vi "TestArrays.vi"() -> ()   [LabVIEW 2010]
panel:
  in  "Array":u32[](array[numeric])
  out "Numeric 10":i32
  out "Numeric 9":i32
  out "Numeric 8":i32
  out "Numeric 7":i32
  out "Numeric 6":i32
  out "Numeric 5":i32
  out "Numeric 4":i32
  out "Numeric 3":i32
  out "Numeric 2":i32
  out "Numeric":i32
  out "element":dbl format="%.2f"
  in  "Array Size":i32
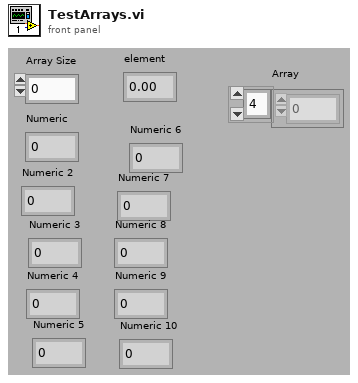
[diagram p1: front panel]
types:
  T1 = cluster{i32, i32, i32, i32, i32, i32, i32, i32, i32, i32}
  T2 = cluster{"[0]":i32, "[1]":i32, "[2]":i32, "[3]":i32, "[4]":i32, "[5]":i32, "[6]":i32, "[7]":i32, "[8]":i32}
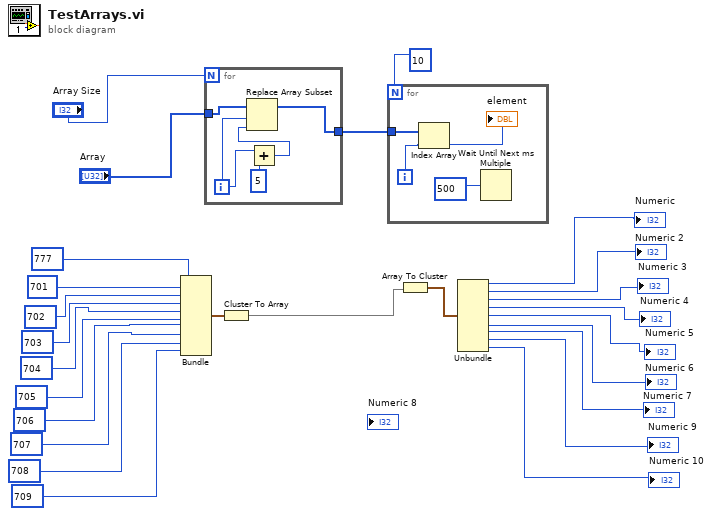
[diagram p0: block diagram]
diagram:
  n1 = Bundle(777, 701, 702, 703, 704, 705, 706, 707, 708, 709) -> (w6:T1)  [unwired: 1 in]
  n2 = for {
    N: "Array Size" -> [_]
    tunnel: "Array" -> [w31]
    tunnel: [w30] -> w2
    i -> [w28]
    n3 = Add(x=w28, y=u32 5) -> (x+y=w27:u32)
    n4 = Replace Array Subset(array=w31, new element=w27, index=w28) -> (w30:u32[])
  }
  n5 = Cluster To Array(cluster=w6) -> (array=w3:i32[])
  n6 = for {
    N: 10 -> [_]
    tunnel: w2 -> [w33]
    i -> [w35]
    n7 = Index Array(array=w33, index=w35) -> (element=→"element":u32)
    n8 = Wait Until Next ms Multiple(millisecond multiple=500) -> ()  [unwired: 1 out]
  }
  n9 = Array To Cluster(array=w3) -> (cluster=w26:T2)
  n10 = Unbundle(w26) -> ("[0]"=→"Numeric":i32, "[1]"=→"Numeric 2":i32, "[2]"=→"Numeric 3":i32, "[3]"=→"Numeric 4":i32, "[4]"=→"Numeric 5":i32, "[5]"=→"Numeric 6":i32, "[6]"=→"Numeric 7":i32, "[7]"=→"Numeric 9":i32, "[8]"=→"Numeric 10":i32)
